vi "Screen_MainScreen.vi"() -> ()   [LabVIEW 2013]
uses:
  Autotest.ctl
  030 - EVENTS/EnumFgvEventCommand.ctl
  MainScreen_AppContext.ctl
  030 - EVENTS/03 - ToMessageHandlerProcess/ToMessageHandlerEvent.ctl
  030 - EVENTS/03 - ToMessageHandlerProcess/enumMessageCriticity.ctl
  090 - ERRORS/Ctrls/enumLogAndView.ctl
  enumScreen.ctl
  SubVis/Ctrls/EnumLockUnlockScreen.ctl
panel:
  in  "Bouton Test 2":bool
  in  "Bouton Test":bool
  in  "Bouton Configuration":bool
  out "Logo 400 X 400":picture
  in  "Autotest results":i32(listbox)
  in  "Autotest":T1
  in  "Bouton Traduction":bool
  in  "Bouton Visualisation LOG":bool
  in  "Bouton Quitter":bool
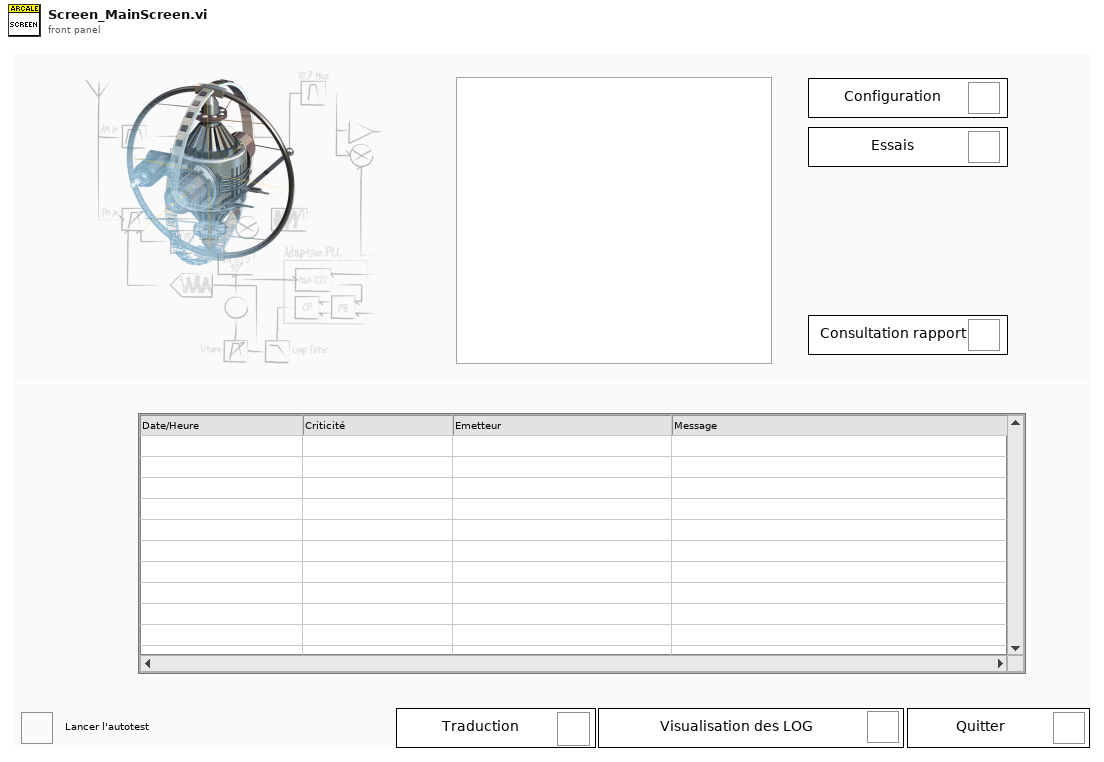
[diagram p1: front panel]
types:
  T1 = typedef "Autotest.ctl" = bool
  T2 = typedef "enumLogAndView.ctl" = enum16{"Log only", "Log and view"}
  T3 = typedef "MainScreen_AppContext.ctl" = cluster{"Number of autotest results":u16, "MessageArray":T4[]}
  T4 = typedef "ToMessageHandlerEvent.ctl" = cluster{"date / time":timestamp, "Criticity":T5, "Emitter":string, "Message":string}
  T5 = typedef "enumMessageCriticity.ctl" = enum16{"No error", "Info", "Warning", "Error", "Fatal error"}
  T6 = typedef "EnumFgvEventCommand.ctl" = enum16{"Setup", "Cleanup", "Get"}
  T7 = typedef "ApplicationInfos.ctl" = cluster{"ApplicationName":string, "ApplicationVersion":string, "Logo 600X200 path":path, "Logo 400X400 path":path, "Client":string}
  T8 = typedef "enumScreen.ctl" = enum16{"Test screen", "Ecran principal", "LOG", "Setup", "Popup : About", "Popup : View last message", "Popup : WebBrowser help", "Traduction", "Popup : DEBUG Process"}
  T9 = cluster{"date / time":timestamp, "Criticity":T5, "Emitter":string, "Message":string}[]
  T10 = typedef "EnumLockUnlockScreen.ctl" = enum16{"Lock screen", "Unlock screen"}
  T11 = typedef "FromProcessesEventType.ctl" = enum16{"Started", "Autotest", "Ended"}
  T12 = typedef "ToScreensCommand.ctl" = enum16{"Stop screen", "Stop all screens"}
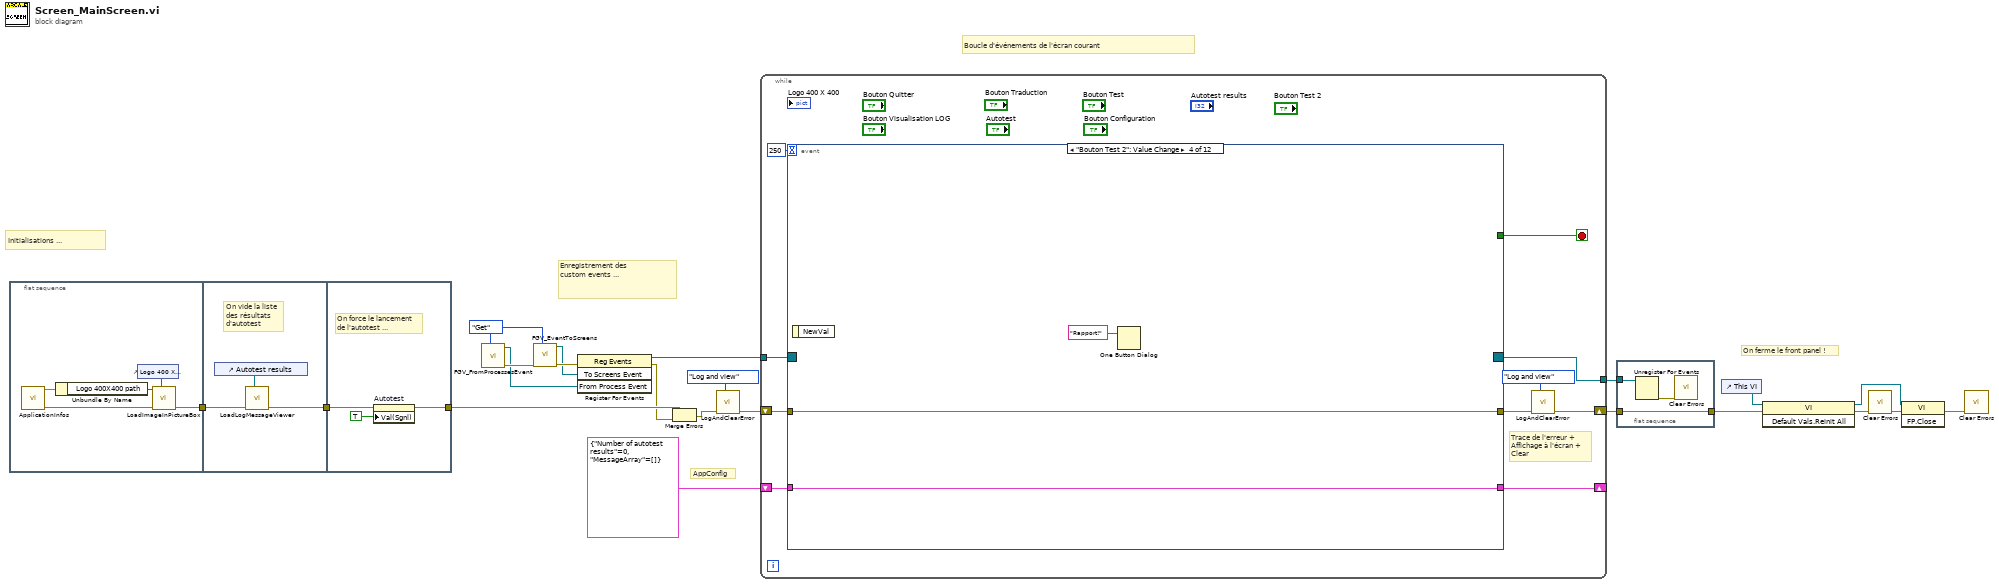
[diagram p0: block diagram]
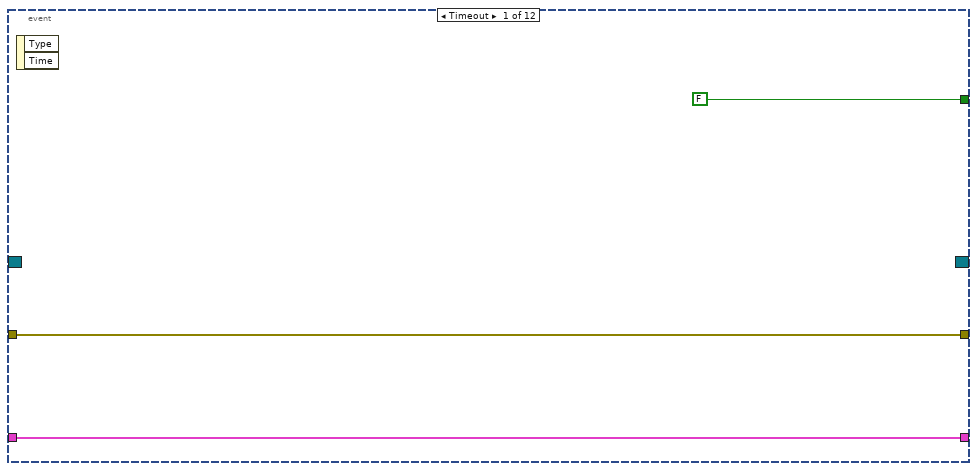
[diagram p2: hidden frame]
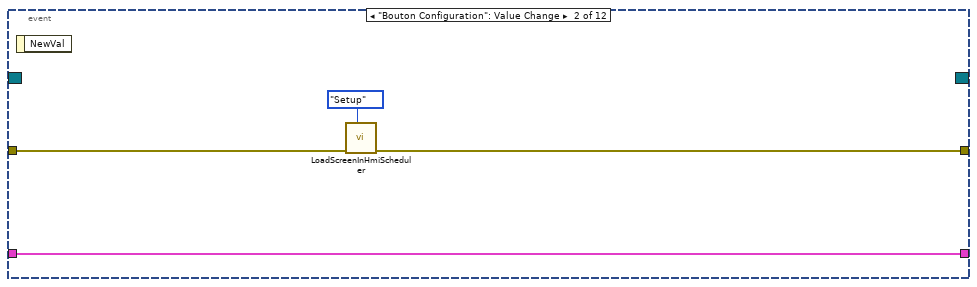
[diagram p3: hidden frame]
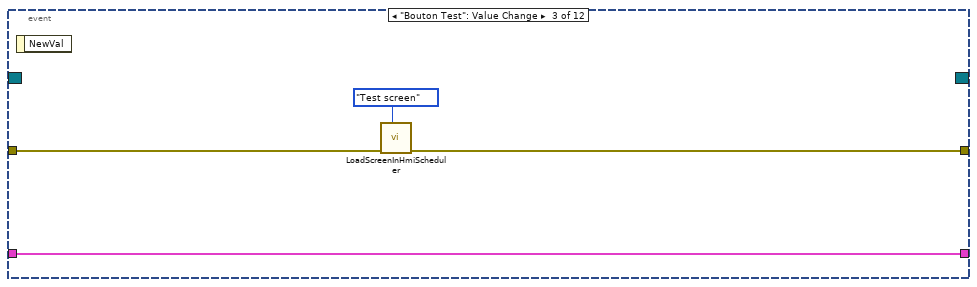
[diagram p4: hidden frame]
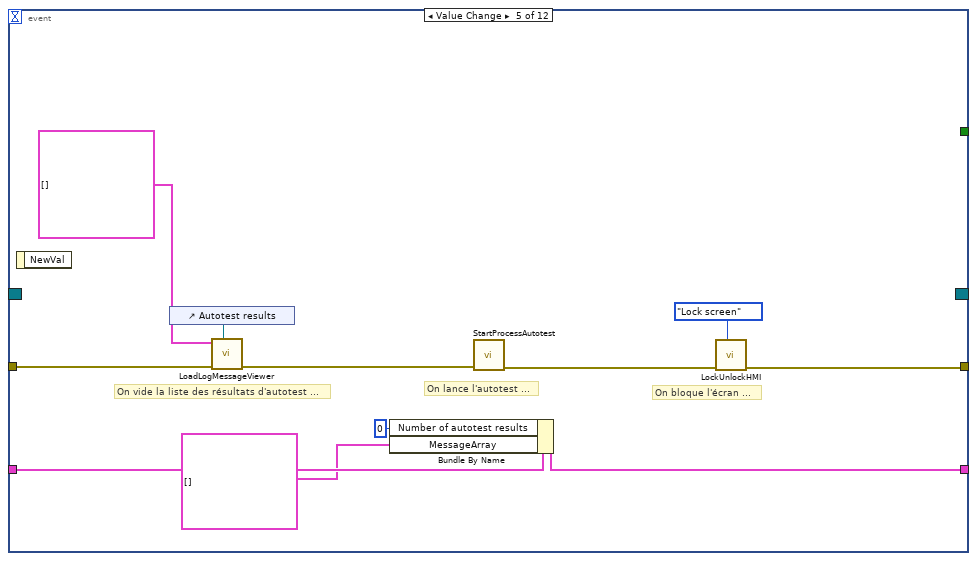
[diagram p5: hidden frame]
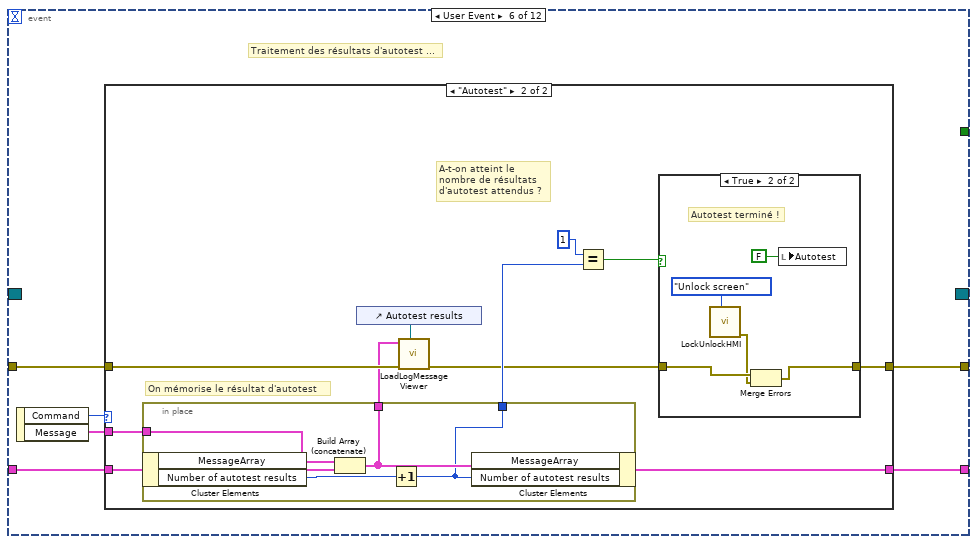
[diagram p6: hidden frame]
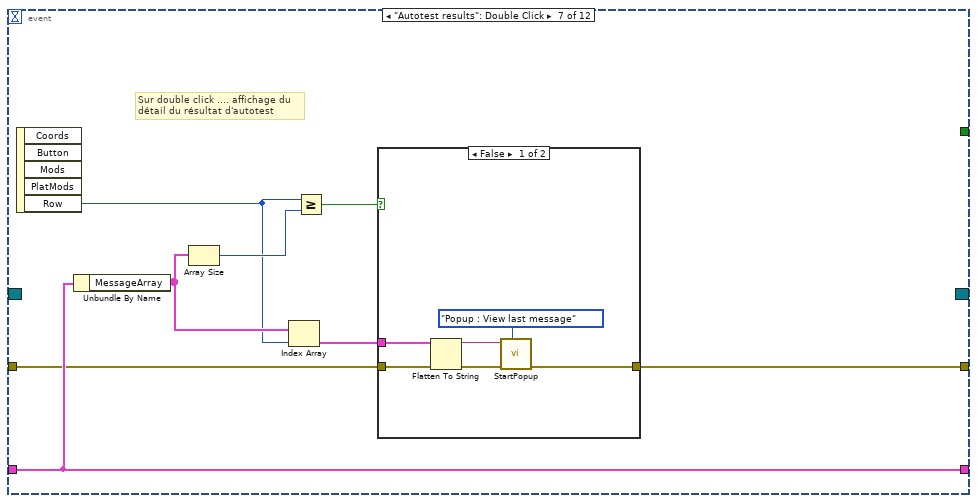
[diagram p9: hidden frame]
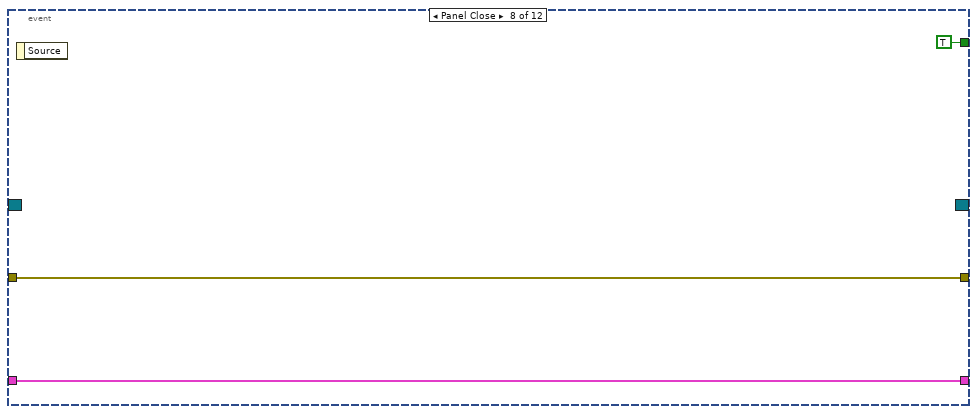
[diagram p11: hidden frame]
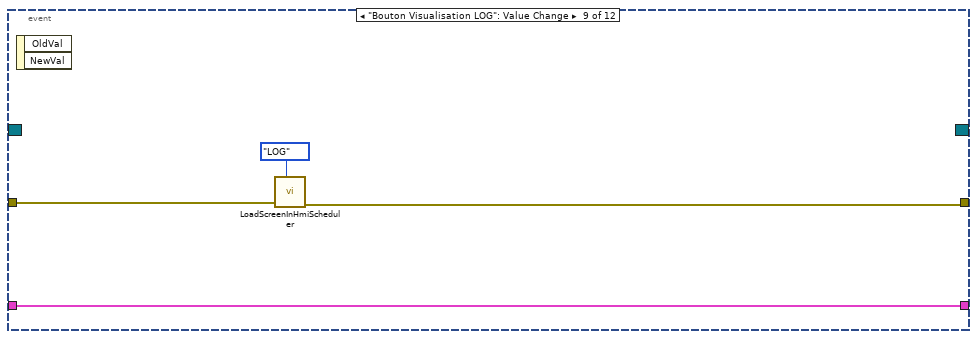
[diagram p12: hidden frame]
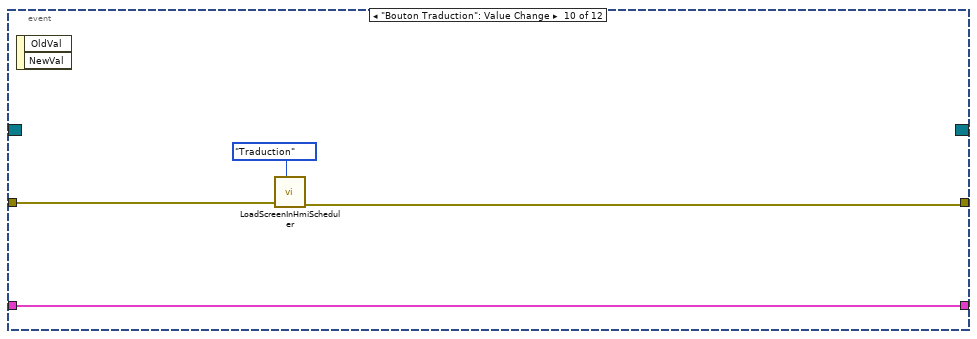
[diagram p13: hidden frame]
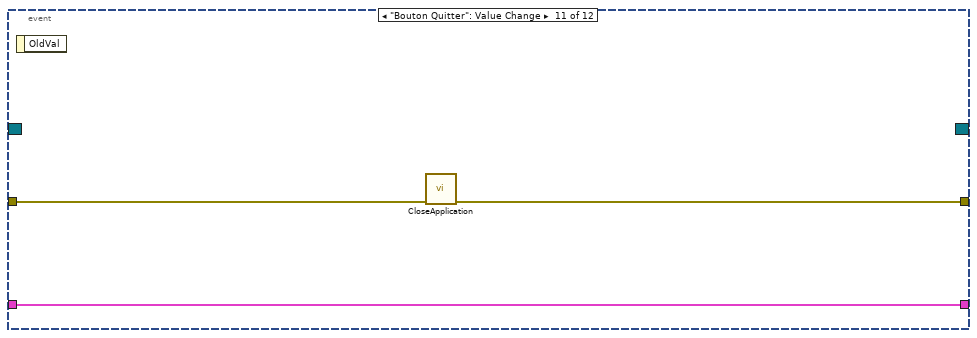
[diagram p14: hidden frame]
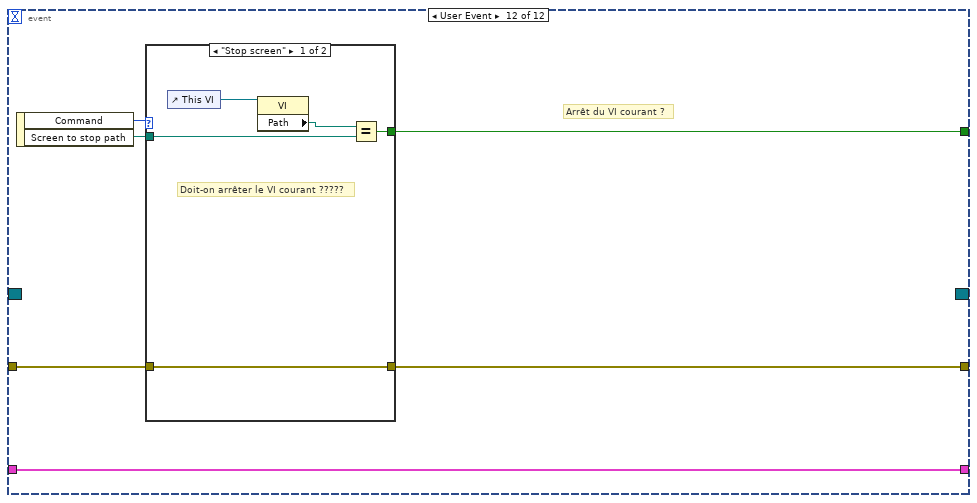
[diagram p15: hidden frame]
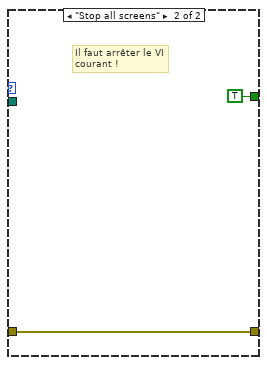
[diagram p16: hidden frame]
diagram:
  w9 = EnumFgvEventCommand."Get" ("Command")
  # "Initialisations ..."
  # "AppConfig"
  # "Enregistrement des\ncustom events ..."
  # "On ferme le front panel !"
  # "Boucle d'événements de l'écran courant"
  n1 = flat-sequence {
    tunnel: [w25] -> w11
    tunnel: w11 -> [w29]
    tunnel: [w28] -> w7
    tunnel: [w31] -> w13
    tunnel: w7 -> [w32]
    frame #0 {
      n2 = call "ApplicationInfos.vi"() -> ("error out"=w23:errorcluster, "ApplicationInfo"=w26:T7)  [unwired: 10 in]
      n3 = Unbundle By Name(w26) -> ("Logo 400X400 path"=w24:path)
      n4 = control-ref of="Logo 400 X 400"() -> (w27:refnum<vi>)
      n5 = call "LoadImageInPictureBox.vi"("Pict Refnum In"=w27, "error in (no error)"=w23, "Image file path"=w24) -> ("error out"=w25:errorcluster)  [unwired: 8 in]
    }
    frame #1 {
      # "On vide la liste\ndes résultats \nd'autotest"
      n6 = control-ref of="Autotest results"() -> (w30:refnum<vi>)
      n7 = call "LoadLogMessageViewer.vi"("Messages viewer"=w30, "error In"=w29) -> ("error out"=w28:errorcluster)  [unwired: 9 in]
    }
    frame #2 {
      # "On force le lancement\nde l'autotest ..."
      n8 = property on="Autotest" class="Bool (strict)"(error in=w32, "Val(Sgnl)"=TRUE ("Value (Signaling)")) -> (error out=w31:errorcluster)  [unwired: 1 in, 1 out]
    }
  }
  n9 = call "FGV_FromProcessesEvent.vi"("Command"=w9) -> ("error out"=w10:errorcluster, "From Process Event"=w8:refnum<user-event>)  [unwired: 9 in]
  n10 = call "FGV_EventToScreens.vi"("Command"=w9, "error in (no error)"=w10) -> ("error out"=w22:errorcluster, "To Screens Event"=w21:refnum<user-event>)  [unwired: 8 in]
  n11 = register-events(error in=w22, w21, w8) -> (reference out=w20:refnum<event-registration>, error out=w12:errorcluster)  [unwired: 1 in]
  n12 = Merge Errors(w13, w12) -> (w5:errorcluster)
  n13 = call "LogAndClearError.vi"("Log and view ?"=enumLogAndView."Log and view", "error in (no error)"=w5) -> ("error out"=w4:errorcluster)  [unwired: 9 in]
  n14 = while {
    tunnel: w20 -> [w43]
    shift-right: [w37] -> w18
    shift-left: w4 -> [w42]
    tunnel: [w41] -> w19
    shift-right: [w38] -> _
    shift-left: T3 {"Number of autotest results"=0, "MessageArray"=[]} ("appContext") -> [w39]
    stop <- w40 stop-if-true
    # "Trace de l'erreur +\nAffichage à l'écran +\nClear"
    n15 = event shown="[3] \"Bouton Test 2\": Value Change" {
      selector: w43 -> [_ _ _ _ _ _ _ _ _ _ _ _]
      dyn-events: [_ _ _ _ _ _ _ _ _ _ _ _] -> w41
      timeout: 250 -> [_ _ _ _ _ _ _ _ _ _ _ _]
      tunnel: w42 -> [w46 w49 w53 w57 w67 w72 w103 w116 w119 w123 w127 w132]
      tunnel: [w46 w48 w52 w57 w63 w69 w102 w116 w118 w122 w126 w131] -> w36
      tunnel: [FALSE _ _ _ _ _ _ TRUE _ _ _ w129] -> w40
      tunnel: w39 -> [w44 w47 w51 w56 w61 w71 w106 w115 w117 w121 w125 w128]
      tunnel: [w44 w47 w51 w56 w60 w70 w106 w115 w117 w121 w125 w128] -> w38
      event Timeout {
        n16 = event-data() -> ()  [unwired: 1 in, 2 out]
      }
      event "Bouton Configuration": Value Change {
        n17 = event-data() -> ()  [unwired: 1 in, 1 out]
        n18 = call "LoadScreenInHmiScheduler.vi"("Enum Screen"=enumScreen."Setup", "error in (no error)"=w49) -> ("error out"=w48:errorcluster)  [unwired: 9 in]
      }
      event "Bouton Test": Value Change {
        n19 = event-data() -> ()  [unwired: 1 in, 1 out]
        n20 = call "LoadScreenInHmiScheduler.vi"("Enum Screen"=enumScreen."Test screen", "error in (no error)"=w53) -> ("error out"=w52:errorcluster)  [unwired: 9 in]
      }
      event "Bouton Test 2": Value Change {
        n21 = event-data() -> ()  [unwired: 1 in, 1 out]
        n22 = One Button Dialog(message="Rapport!") -> ()  [unwired: 1 in, 1 out]
      }
      event Value Change {
        # "On bloque l'écran ..."
        # "On lance l'autotest ..."
        # "On vide la liste des résultats d'autotest ..."
        n23 = event-data() -> ()  [unwired: 1 in, 1 out]
        n24 = control-ref of="Autotest results"() -> (w68:refnum<vi>)
        n25 = call "LoadLogMessageViewer.vi"("Messages viewer"=w68, "error In"=w67, "MessageArray"=T4[] []) -> ("error out"=w65:errorcluster)  [unwired: 8 in]
        n26 = Bundle By Name(cluster=w61, "Number of autotest results"=u16 0, "MessageArray"=T9 []) -> (w60:T3)
        n27 = call "StartProcessAutotest.vi"("error in (no error)"=w65) -> ("error out"=w64:errorcluster)  [unwired: 10 in]
        n28 = call "LockUnlockHMI.vi"("Lock / unlock screen ?"=EnumLockUnlockScreen."Lock screen", "error in (no error)"=w64) -> ("error out"=w63:errorcluster)  [unwired: 9 in]
      }
      event User Event {
        # "Traitement des résultats d'autotest ..."
        n29 = event-data() -> ("Command"=w74:T11, "Message"=w73:T4)  [unwired: 1 in]
        n30 = case shown="\"Autotest\"" w74 {
          tunnel: w73 -> [_ w85]
          tunnel: w72 -> [w75 w83]
          tunnel: w71 -> [w76 w87]
          tunnel: [w76 w86] -> w70
          tunnel: [w75 w77] -> w69
          frame Default {
          }
          frame "Autotest" {
            # "A-t-on atteint le\nnombre de résultats\nd'autotest attendus ?"
            # "On mémorise le résultat d'autotest"
            n31 = in-place {
              in-place-border: w85 -> [w96]
              in-place-border: [w95] -> w82
              in-place-border: [w94] -> w81
              n32 = in-place-cluster #1(w87) -> ("MessageArray"=w97:T4[], "Number of autotest results"=w98:u16)
              n33 = Build Array (concatenate)(w97, w96) -> (w95:T4[])
              n34 = Increment(x=w98) -> (x+1=w94:u16)
              n35 = in-place-cluster #1("MessageArray"=w95, "Number of autotest results"=w94) -> (w86:T3)
            }
            n36 = control-ref of="Autotest results"() -> (w84:refnum<vi>)
            n37 = call "LoadLogMessageViewer.vi"("Messages viewer"=w84, "error In"=w83, "MessageArray"=w82) -> ("error out"=w78:errorcluster)  [unwired: 8 in]
            n38 = Equal?(x=u16 1, y=w81) -> (x = y?=w79:bool)
            n39 = case shown="True" w79 {
              tunnel: w78 -> [w88 w92]
              tunnel: [w88 w90] -> w77
              frame False {
                # "Autotest en cours ..."
              }
              frame True {
                # "Autotest terminé !"
                n40 = call "LockUnlockHMI.vi"("Lock / unlock screen ?"=EnumLockUnlockScreen."Unlock screen") -> ("error out"=w91:errorcluster)  [unwired: 10 in]
                n41 = Merge Errors(w92, w91) -> (w90:errorcluster)
                n42 = local write "Autotest"(T1 FALSE ("Autotest")) -> ()
              }
            }
          }
        }
      }
      event "Autotest results": Double Click {
        # "Sur double click .... affichage du\ndétail du résultat d'autotest"
        n43 = event-data() -> ("Row"=w99:i32)  [unwired: 1 in, 4 out]
        n44 = Unbundle By Name(w106) -> ("MessageArray"=w100:T4[])
        n45 = Array Size(array=w100) -> (size(s)=w105:i32)
        n46 = Index Array(array=w100, index=w99) -> (element=w101:T4)
        n47 = Greater Or Equal?(x=w99, y=w105) -> (x >= y?=w104:bool)
        n48 = case shown="False" w104 {
          tunnel: w103 -> [w109 w113]
          tunnel: [w108 w113] -> w102
          tunnel: w101 -> [w107 _]
          frame False {
            n49 = Flatten To String(anything=w107, error in (no error)=w109) -> (data string=w110:string, error out=w111:errorcluster)  [unwired: 2 in, 1 out]
            n50 = call "StartPopup.vi"("Popup"=enumScreen."Popup : View last message", "error in (no error)"=w111, "String parameter"=w110) -> ("error out"=w108:errorcluster)  [unwired: 8 in]
          }
          frame True {
          }
        }
      }
      event Panel Close {
        n51 = event-data() -> ()  [unwired: 1 in, 1 out]
      }
      event "Bouton Visualisation LOG": Value Change {
        n52 = event-data() -> ()  [unwired: 1 in, 2 out]
        n53 = call "LoadScreenInHmiScheduler.vi"("Enum Screen"=enumScreen."LOG", "error in (no error)"=w119) -> ("error out"=w118:errorcluster)  [unwired: 9 in]
      }
      event "Bouton Traduction": Value Change {
        n54 = event-data() -> ()  [unwired: 1 in, 2 out]
        n55 = call "LoadScreenInHmiScheduler.vi"("Enum Screen"=enumScreen."Traduction", "error in (no error)"=w123) -> ("error out"=w122:errorcluster)  [unwired: 9 in]
      }
      event "Bouton Quitter": Value Change {
        n56 = event-data() -> ()  [unwired: 1 in, 1 out]
        n57 = call "CloseApplication.vi"("error in (no error)"=w127) -> ("error out"=w126:errorcluster)  [unwired: 10 in]
      }
      event User Event {
        # "Arrêt du VI courant ?"
        n58 = event-data() -> ("Command"=w133:T12, "Screen to stop path"=w130:path)  [unwired: 1 in]
        n59 = case shown="\"Stop screen\"" w133 {
          tunnel: w132 -> [w138 w139]
          tunnel: [w138 w139] -> w131
          tunnel: w130 -> [w135 _]
          tunnel: [w134 TRUE] -> w129
          frame "Stop screen" {
            # "Doit-on arrêter le VI courant ?????"
            n60 = control-ref of="This VI"() -> (w137:refnum<vi>)
            n61 = property class="VI"(reference=w137) -> ("Path"=w136:path)  [unwired: 1 in, 2 out]
            n62 = Equal?(x=w136, y=w135) -> (x = y?=w134:bool)
          }
          frame "Stop all screens" {
            # "Il faut arrêter le VI\ncourant !"
          }
        }
      }
    }
    n63 = call "LogAndClearError.vi"("Log and view ?"=enumLogAndView."Log and view", "error in (no error)"=w36) -> ("error out"=w37:errorcluster)  [unwired: 9 in]
  }
  n64 = flat-sequence {
    tunnel: w19 -> [w143]
    tunnel: w18 -> [w141]
    tunnel: [w141] -> w16
    frame #0 {
      n65 = Unregister For Events(event registration refnum=w143) -> (error out=w142:errorcluster)  [unwired: 1 in]
      n66 = call <vilib>:"Clear Errors.vi"("error in (no error)"=w142) -> ()  [unwired: 6 in, 1 out]
    }
  }
  n67 = control-ref of="This VI"() -> (w15:refnum<vi>)
  n68 = invoke class="VI" method="Default Vals.Reinit All"(reference=w15, error in=w16) -> (reference out=w1:refnum<vi>, error out=w17:errorcluster)  [unwired: 1 in, 1 out]
  n69 = call <vilib>:"Clear Errors.vi"("error in (no error)"=w17) -> ("error out"=w2:errorcluster)  [unwired: 6 in]
  n70 = invoke class="VI" method="FP.Close"(reference=w1, error in=w2) -> (error out=w3:errorcluster)  [unwired: 1 in, 2 out]
  n71 = call <vilib>:"Clear Errors.vi"("error in (no error)"=w3) -> ()  [unwired: 6 in, 1 out]
